vi "R_METLA_KE2410_CommandsGlobal.vi"() -> ()   [LabVIEW 2019, in "R_Metal_KE2410.lvclass"]
uses:
  R_Metal_KE2410.lvclass
panel:
  in  "R_METAL 2410 GPIB Setup":T1={"Instrument name"="R_Metal Keithley 2410", "Command \"Reset\""="*rst", "Command \"Initialise\""=":Calculate:state 0; :trigger:source imm; :trigger:count 1; :format:data ASCii; :format:elements VOLT; :trace:tstamp:format delta; :source:current:range MIN; :sense:func 'VOLT:DC'; :sense:voltage:range:auto 1; :sense:voltage:prot %1.6f;", "Command \"Arm\""=":outp:stat OFF; :sour:func CURR; :sour:curr:mode FIX; :sour:curr:lev 0; :outp:stat ON; ", "Command \"SetVolts\""=":sour:curr:lev %4.2f; :sense:voltage:range:auto 1; :sense:voltage:prot %1.6f;", "Command \"Compliance?\""=":SENS:VOLT:PROT:TRIP?;", "Command \"Standby\""=":sour:CURR:lev 0.0; :outp:stat OFF;\n", "Command \"Read Current\""="READ?"}
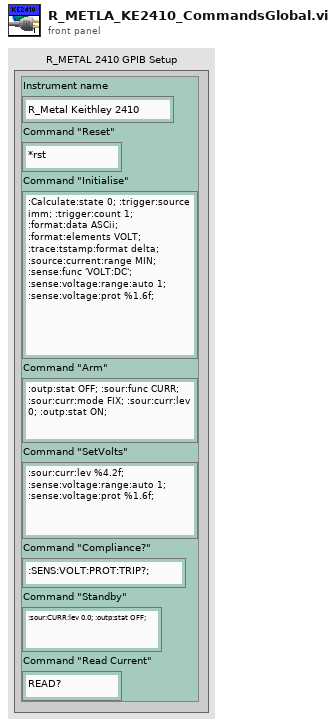
[diagram p1: front panel]
types:
  T1 = cluster{"Instrument name":string, "Command \"Reset\"":string, "Command \"Initialise\"":string, "Command \"Arm\"":string, "Command \"SetVolts\"":string, "Command \"Compliance?\"":string, "Command \"Standby\"":string, "Command \"Read Current\"":string}
diagram:
